vi "Core1.vi"(8 "error in (no error)":errorcluster, 11 "MB in":refnum<class "Master CR.lvclass">) -> (0 "consumer error":errorcluster, 3 "MB out":refnum<class "Master CR.lvclass">)   [LabVIEW 2021, in "Master CR.lvclass"]
uses:
  Master CR.lvclass
  Master CR.lvclass/Master CR.ctl
  ctl/CR_Core_State.ctl
panel:
  out "MHL error":errorcluster
  in  "write enable":bool=TRUE
  out "CR_Core_State":T1=enum."requests"
  in  "stop":bool
  out "stopped":bool
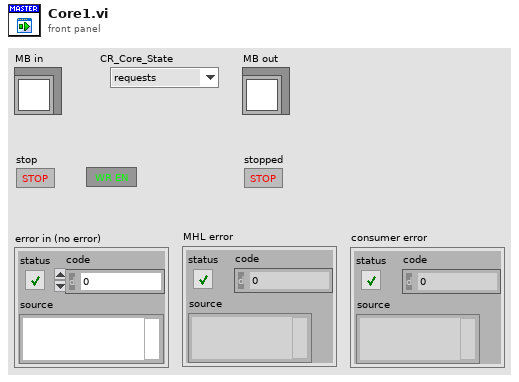
[diagram p1: front panel]
types:
  T1 = typedef "Master CR.lvclass/CR_Core_State.ctl" = enum8{"initialization", "redefine", "standby", "ping", "connect", "wait to reconnect", "wait to reset timeout", "configure", "requests", "close connection", "stop"}
  T2 = typedef "Master CR.lvclass/MB timeouts.ctl" = cluster{"reconn_timeout":i32, "N attempt max":i32, "t_reset_TTL":i32, "period":i32}
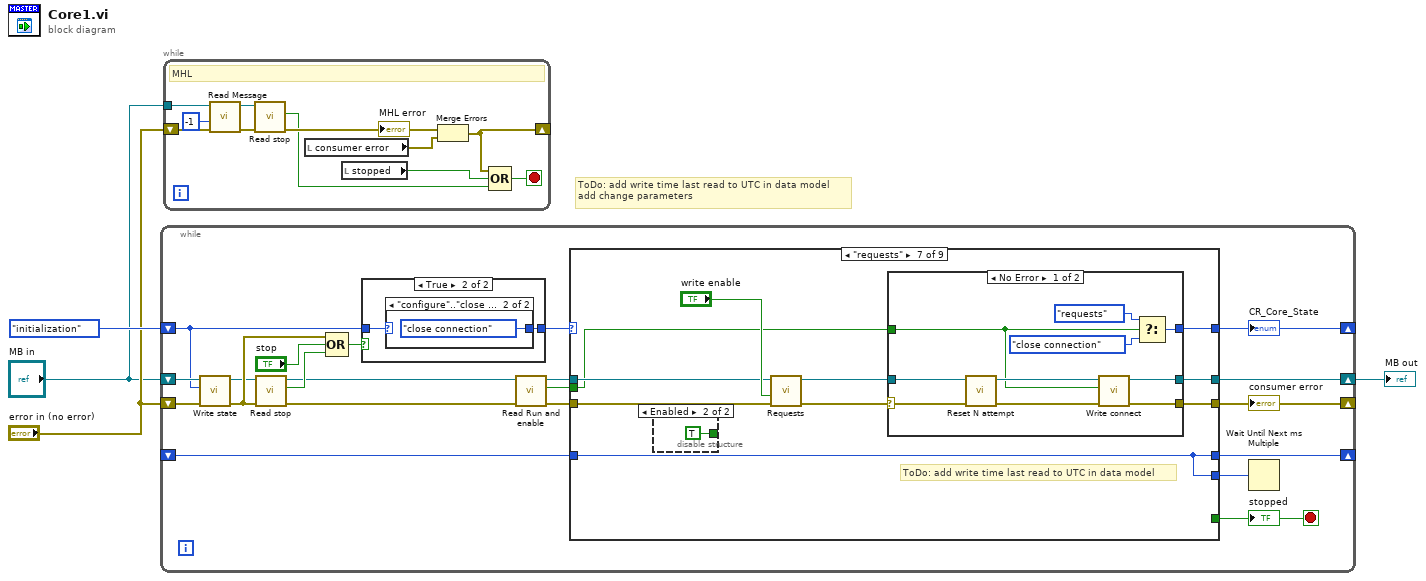
[diagram p0: block diagram]
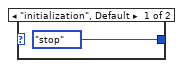
[diagram p3: hidden frame]
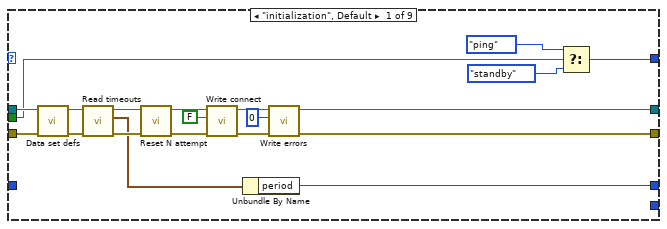
[diagram p4: hidden frame]
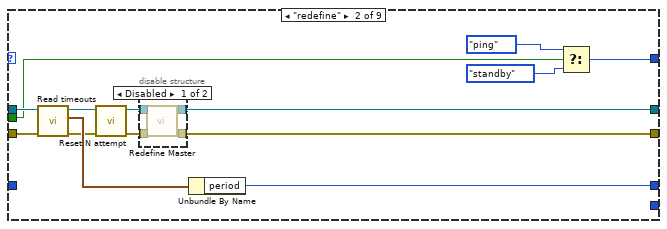
[diagram p5: hidden frame]
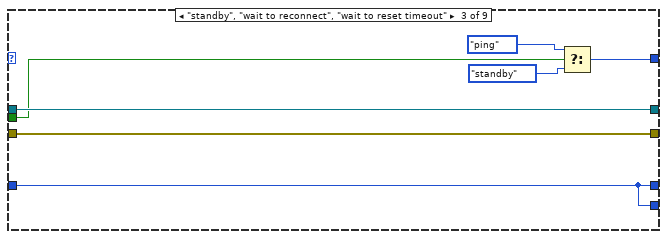
[diagram p7: hidden frame]
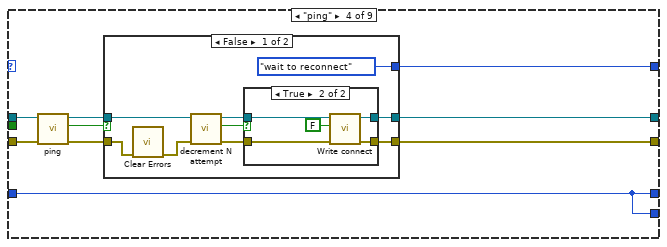
[diagram p8: hidden frame]
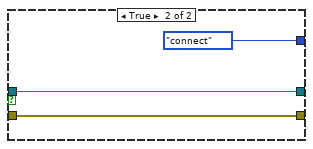
[diagram p10: hidden frame]
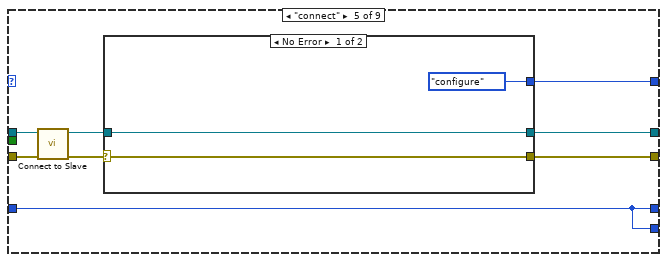
[diagram p11: hidden frame]
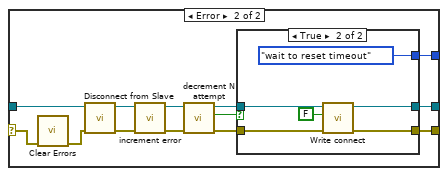
[diagram p12: hidden frame]
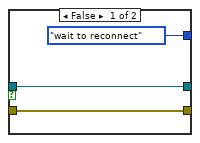
[diagram p13: hidden frame]
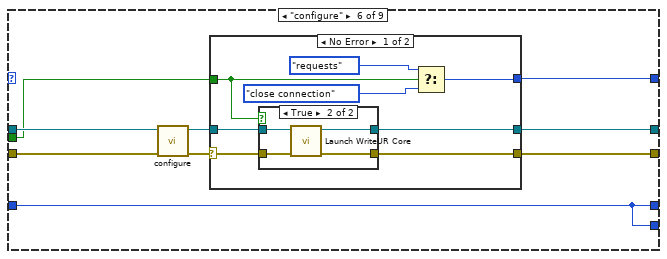
[diagram p14: hidden frame]
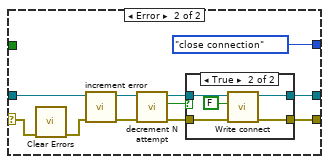
[diagram p16: hidden frame]
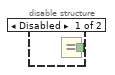
[diagram p18: hidden frame]
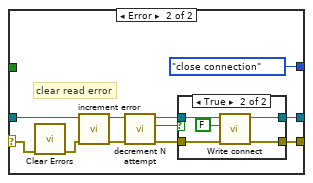
[diagram p19: hidden frame]
diagram:
  # "ToDo: add write time last read to UTC in data model\nadd change parameters"
  n1 = while {
    shift-right: [w22] -> w4
    shift-left: "MB in" -> [w15]
    shift-right: [w20] -> _
    shift-left: "error in (no error)" -> [w14]
    shift-right: [w24] -> _
    shift-left: _ -> [w25]
    shift-right: [w21] -> _
    shift-left: CR_Core_State."initialization" ("state") -> [w6]
    stop <- w19 stop-if-true
    n2 = call "Write state.vi"("error in (no error)"=w14, "state"=w6, "Master CR in"=w15) -> ("error out"=w10:errorcluster, "Master CR out"=w9:refnum<class "Master CR.lvclass">)  [unwired: 7 in]
    n3 = call "Read stop.vi"("error in (no error)"=w10, "Master CR in"=w9) -> ("error out"=w7:errorcluster, "Stop"=w12:bool, "Master CR out"=w8:refnum<class "Master CR.lvclass">)  [unwired: 7 in]
    n4 = Compound Arithmetic op=OR(w10, "stop", w12) -> (w11:bool)
    n5 = case shown="True" w11 {
      tunnel: w6 -> [w26 w28]
      tunnel: [w26 w27] -> w5
      frame False {
      }
      frame True {
        n6 = case shown="\"configure\"..\"close connection\"" w28 {
          tunnel: [CR_Core_State."stop" ("MB_TCP_State") CR_Core_State."close connection" ("MB_TCP_State")] -> w27
          frame "initialization", Default {
          }
          frame "configure".."close connection" {
          }
        }
      }
    }
    n7 = call "Read Run and enable.vi"("error in (no error)"=w7, "Master CR in"=w8) -> ("error out"=w18:errorcluster, "Enable and Run"=w16:bool, "Master CR out"=w17:refnum<class "Master CR.lvclass">)  [unwired: 7 in]
    n8 = case shown="\"requests\"" w5 {
      tunnel: [_ _ _ _ _ _ _ _ TRUE] -> w19
      tunnel: w17 -> [w48 w61 w74 w82 w109 w141 w181 w229 w236]
      tunnel: [w33 w53 w74 w86 w113 w147 w188 w221 w239] -> w22
      tunnel: w18 -> [w49 w60 w73 w81 w110 w140 w180 w228 w235]
      tunnel: [w34 w62 w75 w85 w112 w146 w187 w222 CR_Core_State."initialization" ("MB_TCP_State")] -> w21
      tunnel: [w32 w52 w73 w84 w111 w145 w186 w220 w238] -> w20
      tunnel: [w50 w58 w71 w83 w106 w144 w184 w230 w243] -> w24
      tunnel: w25 -> [_ _ w71 w83 w106 w144 w184 w230 w243]
      tunnel: [_ _ w71 w83 w106 w144 w184 _ _] -> w23
      tunnel: w16 -> [w31 w51 w72 _ _ w139 w179 w219 _]
      frame "initialization", Default {
        n9 = call "Data set defs.vi"("error in (no error)"=w49, "Master CR in"=w48) -> ("error out"=w43:errorcluster, "Master CR out"=w46:refnum<class "Master CR.lvclass">)  [unwired: 8 in]
        n10 = call "Read timeouts.vi"("error in (no error)"=w43, "Master CR in"=w46) -> ("error out"=w47:errorcluster, "MB timeouts"=w44:T2, "Master CR out"=w45:refnum<class "Master CR.lvclass">)  [unwired: 7 in]
        n11 = call "Reset N attempt.vi"("error in (no error)"=w47, "Master CR in"=w45) -> ("error out"=w41:errorcluster, "Master CR out"=w42:refnum<class "Master CR.lvclass">)  [unwired: 8 in]
        n12 = call "Write connect.vi"("error in (no error)"=w41, "connect"=FALSE, "Master CR in"=w42) -> ("error out"=w39:errorcluster, "Master CR out"=w38:refnum<class "Master CR.lvclass">)  [unwired: 7 in]
        n13 = Unbundle By Name(w44) -> ("period"=w50:i32)
        n14 = call "Write errors.vi"("error in (no error)"=w39, "errors"=0, "Master CR in"=w38) -> ("error out"=w32:errorcluster, "Master CR out"=w33:refnum<class "Master CR.lvclass">)  [unwired: 7 in]
        n15 = Select(t=CR_Core_State."ping" ("MB_TCP_State"), s=w31, f=CR_Core_State."standby" ("MB_TCP_State")) -> (s? t:f=w34:T1)
      }
      frame "redefine" {
        n16 = call "Read timeouts.vi"("error in (no error)"=w60, "Master CR in"=w61) -> ("error out"=w57:errorcluster, "MB timeouts"=w59:T2, "Master CR out"=w56:refnum<class "Master CR.lvclass">)  [unwired: 7 in]
        n17 = call "Reset N attempt.vi"("error in (no error)"=w57, "Master CR in"=w56) -> ("error out"=w54:errorcluster, "Master CR out"=w55:refnum<class "Master CR.lvclass">)  [unwired: 8 in]
        n18 = disable-structure shown="Disabled" {
          disable-tunnel: w55 -> [w68 w70]
          disable-tunnel: w54 -> [w67 w69]
          disable-tunnel: [w66 w70] -> w53
          disable-tunnel: [w65 w69] -> w52
          frame Disabled {
            n19 = call "Redefine Master.vi"("error in (no error)"=w67, "Master CR in"=w68) -> ("error out"=w65:errorcluster, "Master CR out"=w66:refnum<class "Master CR.lvclass">)  [unwired: 8 in]
          }
          frame Enabled {
          }
        }
        n20 = Unbundle By Name(w59) -> ("period"=w58:i32)
        n21 = Select(t=CR_Core_State."ping" ("MB_TCP_State"), s=w51, f=CR_Core_State."standby" ("MB_TCP_State")) -> (s? t:f=w62:T1)
      }
      frame "standby", "wait to reconnect", "wait to reset timeout" {
        n22 = Select(t=CR_Core_State."ping" ("MB_TCP_State"), s=w72, f=CR_Core_State."standby" ("MB_TCP_State")) -> (s? t:f=w75:T1)
      }
      frame "ping" {
        n23 = call-dynamic "ping.vi"("error in (no error)"=w81, "MB_TCP in"=w82) -> ("error out"=w78:errorcluster, "Ping OK"=w79:bool, "MB_TCP out"=w80:refnum<class "Master CR.lvclass">)  [unwired: 7 in]
        n24 = case shown="False" w79 {
          tunnel: w80 -> [w89 w105]
          tunnel: [CR_Core_State."wait to reconnect" ("MB_TCP_State") CR_Core_State."connect" ("MB_TCP_State")] -> w85
          tunnel: [w94 w105] -> w86
          tunnel: [w93 w103] -> w84
          tunnel: w78 -> [w90 w103]
          frame False {
            n25 = call <vilib>:"Clear Errors.vi"("error in (no error)"=w90) -> ("error out"=w88:errorcluster)  [unwired: 5 in, 1 out]
            n26 = call "decrement N attempt.vi"("error in (no error)"=w88, "Master CR in"=w89) -> ("error out"=w91:errorcluster, "=0"=w95:bool, "Master CR out"=w92:refnum<class "Master CR.lvclass">)  [unwired: 7 in]
            n27 = case shown="True" w95 {
              tunnel: w92 -> [w97 w99]
              tunnel: [w97 w102] -> w94
              tunnel: w91 -> [w96 w98]
              tunnel: [w96 w100] -> w93
              frame False {
              }
              frame True {
                n28 = call "Write connect.vi"("error in (no error)"=w98, "connect"=FALSE, "Master CR in"=w99) -> ("error out"=w100:errorcluster, "Master CR out"=w102:refnum<class "Master CR.lvclass">)  [unwired: 7 in]
              }
            }
          }
          frame True {
          }
        }
      }
      frame "connect" {
        n29 = call-dynamic "Connect to Slave.vi"("error in (no error)"=w110, "network master in"=w109) -> ("error out"=w107:errorcluster, "network master out"=w108:refnum<class "Master CR.lvclass">)  [unwired: 8 in]
        n30 = case shown="No Error" w107 {
          selector: w107 -> [w114 w121]
          tunnel: w108 -> [w115 w122]
          tunnel: [CR_Core_State."configure" ("MB_TCP_State") w127] -> w112
          tunnel: [w115 w126] -> w113
          tunnel: [w114 w125] -> w111
          frame No Error {
          }
          frame Error {
            n31 = call <vilib>:"Clear Errors.vi"("error in (no error)"=w121) -> ("error out"=w120:errorcluster)  [unwired: 5 in, 1 out]
            n32 = call-dynamic "Disconnect from Slave.vi"("error in (no error)"=w120, "network master in"=w122) -> ("error out"=w123:errorcluster, "network master out"=w124:refnum<class "Master CR.lvclass">)  [unwired: 8 in]
            n33 = call "increment error.vi"("error in (no error)"=w123, "Master CR in"=w124) -> ("error out"=w119:errorcluster, "Master CR out"=w129:refnum<class "Master CR.lvclass">)  [unwired: 7 in, 1 out]
            n34 = call "decrement N attempt.vi"("error in (no error)"=w119, "Master CR in"=w129) -> ("error out"=w117:errorcluster, "=0"=w128:bool, "Master CR out"=w118:refnum<class "Master CR.lvclass">)  [unwired: 7 in]
            n35 = case shown="True" w128 {
              tunnel: [CR_Core_State."wait to reconnect" ("MB_TCP_State") CR_Core_State."wait to reset timeout" ("MB_TCP_State")] -> w127
              tunnel: w118 -> [w131 w134]
              tunnel: [w131 w137] -> w126
              tunnel: w117 -> [w130 w133]
              tunnel: [w130 w135] -> w125
              frame False {
              }
              frame True {
                n36 = call "Write connect.vi"("error in (no error)"=w133, "connect"=FALSE, "Master CR in"=w134) -> ("error out"=w135:errorcluster, "Master CR out"=w137:refnum<class "Master CR.lvclass">)  [unwired: 7 in]
              }
            }
          }
        }
      }
      frame "configure" {
        n37 = call-dynamic "configure.vi"("error in (no error)"=w140, "Master CR in"=w141) -> ("error out"=w142:errorcluster, "Master CR out"=w143:refnum<class "Master CR.lvclass">)  [unwired: 8 in]
        n38 = case shown="No Error" w142 {
          selector: w142 -> [w150 w170]
          tunnel: [w155 CR_Core_State."close connection" ("MB_TCP_State")] -> w146
          tunnel: [w149 w163] -> w145
          tunnel: w143 -> [w151 w162]
          tunnel: [w148 w164] -> w147
          tunnel: w139 -> [w152 _]
          frame No Error {
            n39 = case shown="True" w152 {
              tunnel: w151 -> [w157 w158]
              tunnel: w150 -> [w156 w160]
              tunnel: [w156 w159] -> w149
              tunnel: [w157 w158] -> w148
              frame False {
              }
              frame True {
                n40 = call "Launch WriteUR Core.vi"("error in"=w160, "Master CR"=w158) -> ("error out"=w159:errorcluster)  [unwired: 9 in]
              }
            }
            n41 = Select(t=CR_Core_State."requests" ("MB_TCP_State"), s=w152, f=CR_Core_State."close connection" ("MB_TCP_State")) -> (s? t:f=w155:T1)
          }
          frame Error {
            n42 = call <vilib>:"Clear Errors.vi"("error in (no error)"=w170) -> ("error out"=w161:errorcluster)  [unwired: 5 in, 1 out]
            n43 = call "increment error.vi"("error in (no error)"=w161, "Master CR in"=w162) -> ("error out"=w166:errorcluster, "Master CR out"=w165:refnum<class "Master CR.lvclass">)  [unwired: 7 in, 1 out]
            n44 = call "decrement N attempt.vi"("error in (no error)"=w166, "Master CR in"=w165) -> ("error out"=w167:errorcluster, "=0"=w169:bool, "Master CR out"=w168:refnum<class "Master CR.lvclass">)  [unwired: 7 in]
            n45 = case shown="True" w169 {
              tunnel: w168 -> [w173 w178]
              tunnel: [w173 w177] -> w164
              tunnel: w167 -> [w172 w176]
              tunnel: [w172 w174] -> w163
              frame False {
              }
              frame True {
                n46 = call "Write connect.vi"("error in (no error)"=w176, "connect"=FALSE, "Master CR in"=w178) -> ("error out"=w174:errorcluster, "Master CR out"=w177:refnum<class "Master CR.lvclass">)  [unwired: 7 in]
              }
            }
          }
        }
      }
      frame "requests" {
        # "ToDo: add write time last read to UTC in data model"
        n47 = disable-structure shown="Enabled" {
          disable-tunnel: [w189 TRUE] -> _
          frame Disabled {
            n48 = Equal?() -> (x = y?=w189:bool)  [unwired: 2 in]
          }
          frame Enabled {
          }
        }
        n49 = call-dynamic "Requests.vi"("error in (no error)"=w180, "write enable"="write enable", "MB_TCP in"=w181) -> ("error out"=w183:errorcluster, "MB_TCP out"=w185:refnum<class "Master CR.lvclass">)  [unwired: 7 in]
        n50 = case shown="No Error" w183 {
          selector: w183 -> [w196 w211]
          tunnel: [w200 CR_Core_State."close connection" ("MB_TCP_State")] -> w187
          tunnel: w179 -> [w193 _]
          tunnel: [w191 w207] -> w186
          tunnel: w185 -> [w197 w204]
          tunnel: [w194 w208] -> w188
          frame No Error {
            n51 = call "Reset N attempt.vi"("error in (no error)"=w196, "Master CR in"=w197) -> ("error out"=w192:errorcluster, "Master CR out"=w195:refnum<class "Master CR.lvclass">)  [unwired: 8 in]
            n52 = call "Write connect.vi"("error in (no error)"=w192, "connect"=w193, "Master CR in"=w195) -> ("error out"=w191:errorcluster, "Master CR out"=w194:refnum<class "Master CR.lvclass">)  [unwired: 7 in]
            n53 = Select(t=CR_Core_State."requests" ("MB_TCP_State"), s=w193, f=CR_Core_State."close connection" ("MB_TCP_State")) -> (s? t:f=w200:T1)
          }
          frame Error {
            # "clear read error"
            n54 = call <vilib>:"Clear Errors.vi"("error in (no error)"=w211) -> ("error out"=w203:errorcluster)  [unwired: 5 in, 1 out]
            n55 = call "increment error.vi"("error in (no error)"=w203, "Master CR in"=w204) -> ("error out"=w205:errorcluster, "Master CR out"=w210:refnum<class "Master CR.lvclass">)  [unwired: 7 in, 1 out]
            n56 = call "decrement N attempt.vi"("error in (no error)"=w205, "Master CR in"=w210) -> ("error out"=w206:errorcluster, "=0"=w202:bool, "Master CR out"=w209:refnum<class "Master CR.lvclass">)  [unwired: 7 in]
            n57 = case shown="True" w202 {
              tunnel: w209 -> [w213 w218]
              tunnel: [w213 w217] -> w208
              tunnel: w206 -> [w212 w216]
              tunnel: [w212 w214] -> w207
              frame False {
              }
              frame True {
                n58 = call "Write connect.vi"("error in (no error)"=w216, "connect"=FALSE, "Master CR in"=w218) -> ("error out"=w214:errorcluster, "Master CR out"=w217:refnum<class "Master CR.lvclass">)  [unwired: 7 in]
              }
            }
          }
        }
      }
      frame "close connection" {
        n59 = call-dynamic "Disconnect from Slave.vi"("error in (no error)"=w228, "network master in"=w229) -> ("error out"=w220:errorcluster, "network master out"=w221:refnum<class "Master CR.lvclass">)  [unwired: 8 in]
        n60 = disable-structure shown="Enabled" {
          disable-tunnel: [w231 TRUE] -> w223
          frame Disabled {
            n61 = Equal?() -> (x = y?=w231:bool)  [unwired: 2 in]
          }
          frame Enabled {
          }
        }
        n62 = Select(t=CR_Core_State."wait to reconnect" ("MB_TCP_State"), s=w223, f=CR_Core_State."redefine" ("MB_TCP_State")) -> (s? t:f=w225:T1)
        n63 = Select(t=w225, s=w219, f=CR_Core_State."standby" ("MB_TCP_State")) -> (s? t:f=w222:T1)
      }
      frame "stop" {
        n64 = call "Write connect.vi"("error in (no error)"=w235, "connect"=FALSE, "Master CR in"=w236) -> ("error out"=w234:errorcluster, "Master CR out"=w233:refnum<class "Master CR.lvclass">)  [unwired: 7 in]
        n65 = call "Write stop.vi"("error in (no error)"=w234, "Stop"=FALSE, "Master CR in"=w233) -> ("error out"=w238:errorcluster, "Master CR out"=w239:refnum<class "Master CR.lvclass">)  [unwired: 7 in]
      }
    }
    "CR_Core_State" <- w21
    "consumer error" <- w20
    "stopped" <- w19
    n66 = Wait Until Next ms Multiple(millisecond multiple=w23) -> ()  [unwired: 1 out]
  }
  "MB out" <- w4
  n67 = while {
    tunnel: "MB in" -> [w252]
    shift-right: [w247] -> _
    shift-left: "error in (no error)" -> [w251]
    stop <- w245 stop-if-true
    # "MHL"
    n68 = call "Read Message.vi"("error in (no error)"=w251, "timeout (0)"=-1, "Master CR in"=w252) -> ("error out"=w250:errorcluster, "Master CR out"=w249:refnum<class "Master CR.lvclass">)  [unwired: 6 in, 1 out]
    n69 = call "Read stop.vi"("error in (no error)"=w250, "Master CR in"=w249) -> ("error out"=w248:errorcluster, "Stop"=w246:bool)  [unwired: 7 in, 1 out]
    "MHL error" <- w248
    n70 = local read "consumer error"() -> (w253:errorcluster)
    n71 = local read "stopped"() -> (w244:bool)
    n72 = Merge Errors(w248, w253) -> (w247:errorcluster)
    n73 = Compound Arithmetic op=OR(w247, w244, w246) -> (w245:bool)
  }
